vi "set working directory.vi"(8 "error in (no error)":errorcluster, 11 "dir":string) -> (0 "error out":errorcluster)   [LabVIEW 2019, in "libSimulationControl.lvlib"]
doc: "void set_working_directory(const char* dir);"
uses:
  libSimulationControl.lvlib
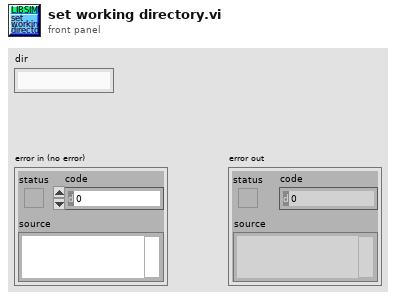
[diagram p1: front panel]
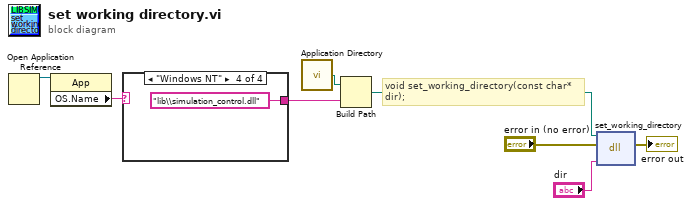
[diagram p0: block diagram]
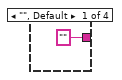
[diagram p2: hidden frame]
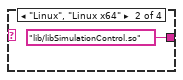
[diagram p3: hidden frame]
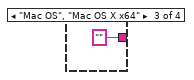
[diagram p4: hidden frame]
diagram:
  # "void set_working_directory(const char* dir);"
  n1 = Open Application Reference() -> (3:w5:refnum<vi>)  [unwired: 4 in, 1 out]
  n2 = property class="App"(reference=w5) -> ("OS.Name"=w4:string)  [unwired: 1 in, 2 out]
  n3 = case shown="\"Windows NT\"" w4 {
    tunnel: ["" ("return type") "lib/libSimulationControl.so" ("name or relative path") "" ("return type") "lib\\simulation_control.dll" ("name or relative path")] -> w3
    frame "", Default {
    }
    frame "Linux", "Linux x64" {
    }
    frame "Mac OS", "Mac OS X x64" {
    }
    frame "Windows NT" {
    }
  }
  n4 = call <vilib>:"Application Directory.vi"() -> ("Application Directory"=w2:path)
  n5 = Build Path(base path=w2, name or relative path=w3) -> (appended path=w1:path)
  n6 = dll-call lib="home/paul/Schreibtisch/Biogas_plant_setup/LabView/lib/libSimulationControl/libSimulationControl.*" fn="set_working_directory"(path in=w1, error in="error in (no error)", "dir"="dir") -> (error out=→"error out":errorcluster)  [unwired: 3 in, 1 out]
